vi "Set VISA Resource.vi"(8 "error in (no error)":errorcluster, 10 "VISA Resource":refnum<visa-resource-name>="COM1", 11 "niDTS Comm Serial in":refnum<class "niDTS Comm Serial.lvclass">) -> (0 "error out":errorcluster, 3 "niDTS Comm Serial out":refnum<class "niDTS Comm Serial.lvclass">)   [LabVIEW 2015, in "niDTS CommLib.lvlib" / "niDTS Comm Serial.lvclass"]
uses:
  niDTS Comm Serial.lvclass
  niDTS Comm Serial.lvclass/niDTS Comm Serial.ctl
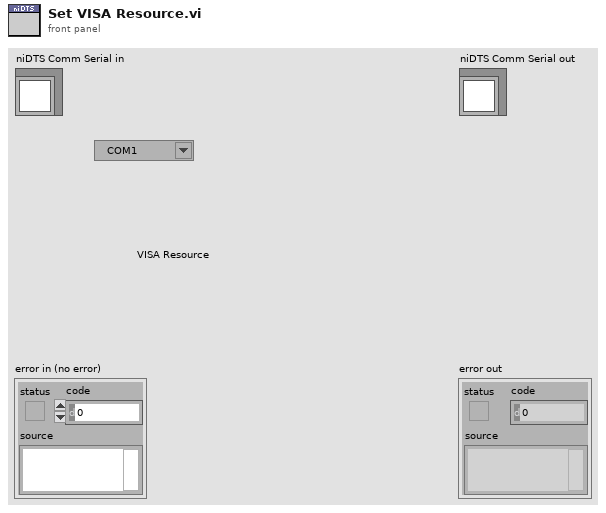
[diagram p1: front panel]
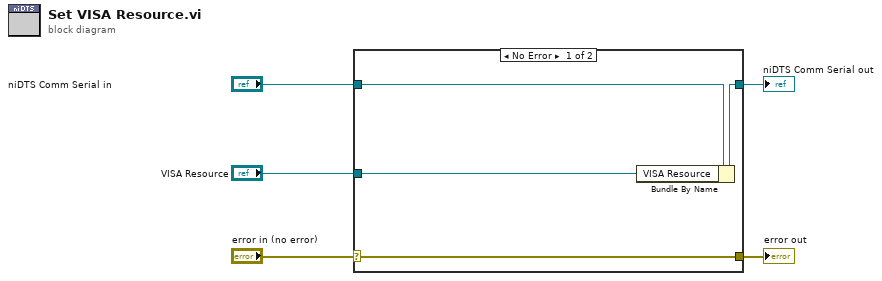
[diagram p0: block diagram]
diagram:
  n1 = case shown="No Error" "error in (no error)" {
    selector: "error in (no error)" -> [w9 w10]
    tunnel: [w9 w10] -> w4
    tunnel: [w7 w11] -> w2
    tunnel: "niDTS Comm Serial in" -> [w8 w11]
    tunnel: "VISA Resource" -> [w6 _]
    frame No Error {
      n2 = Bundle By Name(cluster=w8, "VISA Resource"=w6) -> (w7:refnum<class "niDTS Comm Serial.lvclass">)
    }
    frame Error {
    }
  }
  "error out" <- w4
  "niDTS Comm Serial out" <- w2
